vi "ME Button.vi"() -> (3 "MenuOutput":string)   [LabVIEW 2023]
uses:
  Controls/DisplayQCommand.ctl
  Controls/DisplayMessage.ctl
panel:
  in  "ME":bool
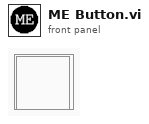
[diagram p1: front panel]
types:
  T1 = typedef "DisplayMessage.ctl" = enum16{"No Message - Ignore", "Display Message", "Set Tab", "Set Status", "Add Error Message", "Clear Error History", "Generate Error", "Set Idling Display", "Set Running Display", "Set Subpanel Output", "Stop"}
  T2 = typedef "DisplayQCommand.ctl" = enum16{"No Command - Error", "Initialise", "Get Q Reference", "Add Item to Bottom", "Add Item to Top", "Flush Q", "Dequeue", "Peek Next Element", "Close"}
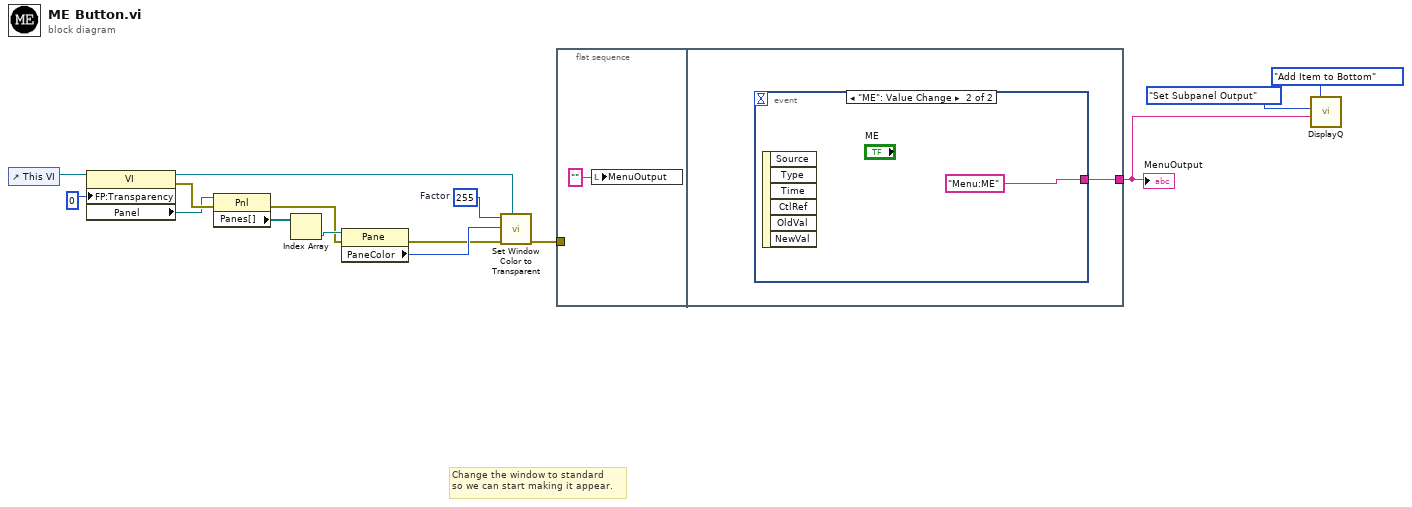
[diagram p0: block diagram]
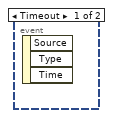
[diagram p2: hidden frame]
diagram:
  w12 = u8 255  # Factor
  # "Change the window to standard\nso we can start making it appear."
  n1 = control-ref of="This VI"() -> (w8:refnum<vi>)
  n2 = property class="VI"(reference=w8, "FP:Transparency"=u8 0 ("t")) -> (reference out=w11:refnum<vi>, error out=w7:errorcluster, "Panel"=w6:refnum<vi>)  [unwired: 1 in]
  n3 = property class="Pnl"(reference=w6, error in=w7) -> (error out=w2:errorcluster, "Panes[]"=w5:refnum<vi>[])  [unwired: 1 out]
  n4 = Index Array(array=w5) -> (element=w4:refnum<vi>)  [unwired: 1 in]
  n5 = property class="Pane"(reference=w4, error in=w2) -> (error out=w1:errorcluster, "PaneColor"=w3:u32)  [unwired: 1 out]
  n6 = call "Set Window Color to Transparent.vi"("Calling VI's reference"=w11, "error in (no error)"=w1, "Color to Replace"=w3, "Factor"=w12) -> ("error out"=w9:errorcluster)  [unwired: 4 in]
  n7 = flat-sequence {
    tunnel: w9 -> [_]
    tunnel: [w17] -> w14
    frame #0 {
      n8 = local write "MenuOutput"("" ("MenuOutput")) -> ()
    }
    frame #1 {
      n9 = event shown="[1] \"ME\": Value Change" {
        selector: _ -> [_ _]
        dyn-events: _ -> [_ _]
        timeout: _ -> [_ _]
        tunnel: [_ "Menu:ME"] -> w17
        event Timeout {
          n10 = event-data() -> ()  [unwired: 1 in, 3 out]
        }
        event "ME": Value Change {
          n11 = event-data() -> ()  [unwired: 1 in, 6 out]
        }
      }
    }
  }
  n12 = call "DisplayQ.vi"("command"=DisplayQCommand."Add Item to Bottom", "DataIn"=w14, "DisplayMessage"=DisplayMessage."Set Subpanel Output") -> ()  [unwired: 2 in, 4 out]
  "MenuOutput" <- w14
